vi "Find next car wash step.vi"(8 "error in (no error)":errorcluster, 11 "Control Refnum":refnum<vi>) -> (0 "error out":errorcluster, 3 "Next Car Wash option":T1)   [LabVIEW 2024]
uses:
  Controls/States.ctl
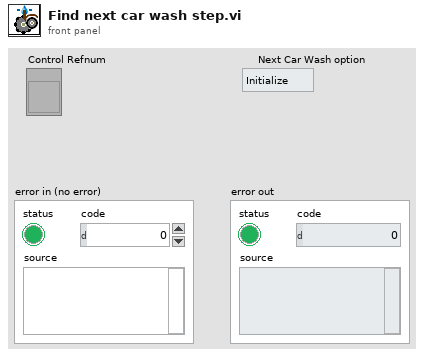
[diagram p1: front panel]
types:
  T1 = typedef "States.ctl" = enum16{"Initialize", "Wait for Event", "Under Body Wash", "Bug Remover", "Pre-Soak", "High Pressure Wash", "Low Pressure Wax", "Spot Free Rinse", "Tire Shine Foam", "Exit", "Air Dry", "Stop"}
  T2 = typedef "Wash Options.ctl" = cluster{"Underbody Wash":bool, "Bug Remover":bool, "Pre-Soak":bool, "High Pressure Wash":bool, "Low Pressure Wax":bool, "Spot Free Rinse":bool, "Tire Shine Foam":bool, "Air Dry":bool}
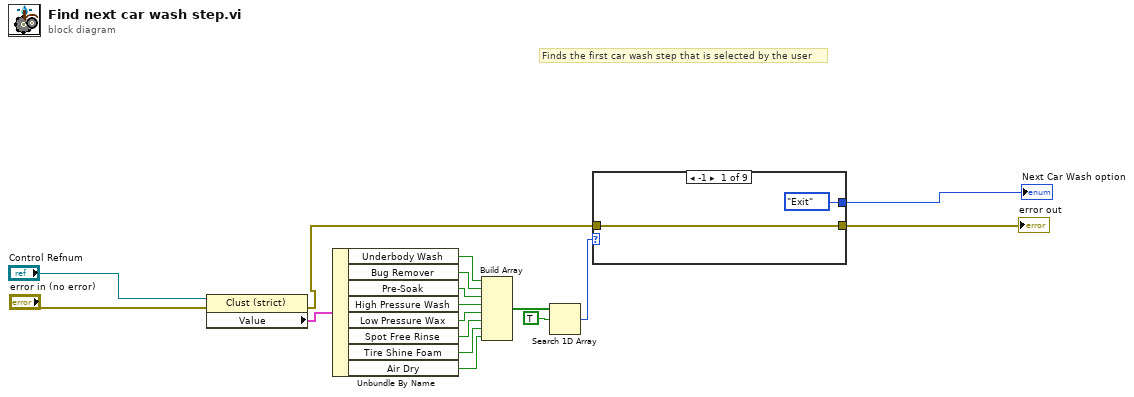
[diagram p0: block diagram]
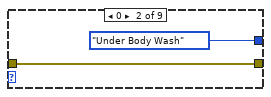
[diagram p2: hidden frame]
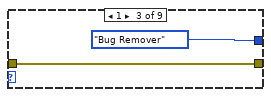
[diagram p3: hidden frame]
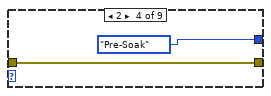
[diagram p4: hidden frame]
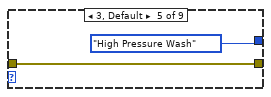
[diagram p5: hidden frame]
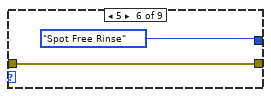
[diagram p6: hidden frame]
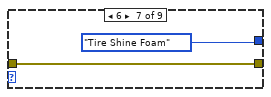
[diagram p7: hidden frame]
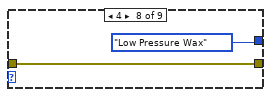
[diagram p8: hidden frame]
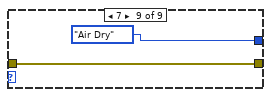
[diagram p9: hidden frame]
diagram:
  # "Finds the first car wash step that is selected by the user"
  n1 = property class="Clust (strict)"(reference="Control Refnum", error in="error in (no error)") -> (error out=w2:errorcluster, "Value"=w4:T2)  [unwired: 1 out]
  n2 = Unbundle By Name(w4) -> ("Underbody Wash"=w6:bool, "Bug Remover"=w7:bool, "Pre-Soak"=w8:bool, "High Pressure Wash"=w9:bool, "Low Pressure Wax"=w10:bool, "Spot Free Rinse"=w11:bool, "Tire Shine Foam"=w12:bool, "Air Dry"=w13:bool)
  n3 = Build Array(w6, w7, w8, w9, w10, w11, w12, w13) -> (w15:bool[])
  n4 = Search 1D Array(1D array=w15, element=TRUE) -> (index of element=w16:i32)  [unwired: 1 in]
  n5 = case shown="-1" w16 {
    tunnel: w2 -> [w18 w21 w23 w25 w27 w29 w31 w33 w35]
    tunnel: [w18 w21 w23 w25 w27 w29 w31 w33 w35] -> w17
    tunnel: [States."Exit" States."Under Body Wash" States."Bug Remover" States."Pre-Soak" States."High Pressure Wash" States."Spot Free Rinse" States."Tire Shine Foam" States."Low Pressure Wax" States."Air Dry"] -> w5
    frame -1 {
    }
    frame 0 {
    }
    frame 1 {
    }
    frame 2 {
    }
    frame 3, Default {
    }
    frame 5 {
    }
    frame 6 {
    }
    frame 4 {
    }
    frame 7 {
    }
  }
  "error out" <- w17
  "Next Car Wash option" <- w5
